vi "Results to Waveforms (array of U8).vi"(1 "data type":u8[][](array[numeric]), 7 "result references":T1[](array[typedef]), 11 "error in (no error)":errorcluster) -> (6 "signals out":u8[][](array[numeric]), 8 "result references out":T1[](array[typedef]), 15 "error out":errorcluster)   [LabVIEW 2020, in "NI_DataFinder.lvlib"]
doc: "Extracts the signals from the results of a DataFinder search."
uses:
  <vilib>/DataFinder/NI_DataFinder.lvlib
  <vilib>/userdefined/DFSearchResult.ctl
  <vilib>/userdefined/NI_DataFinder Controls.lvlib
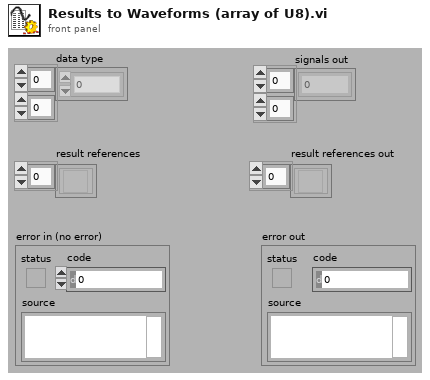
[diagram p1: front panel]
types:
  T1 = typedef "NI_DataFinder Controls.lvlib/DFSearchResult.ctl" = refnum<k20>
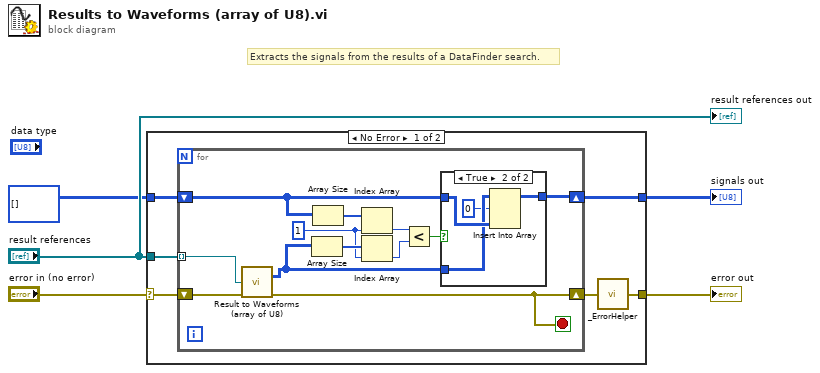
[diagram p0: block diagram]
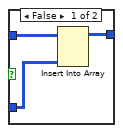
[diagram p2: hidden frame]
diagram:
  # "Extracts the signals from the results of a DataFinder search."
  n1 = case shown="No Error" "error in (no error)" {
    selector: "error in (no error)" -> [w6 w31]
    tunnel: "result references" -> [w11 _]
    tunnel: [w10 w32] -> w4
    tunnel: [w9 w31] -> w3
    tunnel: u8[][] [] ("signals out") -> [w8 w32]
    frame No Error {
      n2 = for {
        shift-right: [w15] -> w10
        shift-left: w8 -> [w14]
        tunnel: w11 -> [w23] mode=indexing
        shift-right: [w12] -> w7
        shift-left: w6 -> [w22]
        stop <- w12 stop-if-true
        w19 = 1 ("index")
        n3 = call <vilib>:"Result to Waveforms (array of U8).vi"("result reference"=w23, "error in"=w22) -> ("signals out"=w13:u8[][], "error out"=w12:errorcluster)  [unwired: 11 in, 1 out]
        n4 = Array Size(array=w13) -> (size(s)=w20:i32[])
        n5 = Array Size(array=w14) -> (size(s)=w21:i32[])
        n6 = Index Array(array=w21, index=w19) -> (element=w17:i32)
        n7 = Index Array(array=w20, index=w19) -> (element=w18:i32)
        n8 = Less?(x=w17, y=w18) -> (x < y?=w16:bool)
        n9 = case shown="True" w16 {
          tunnel: w14 -> [w25 w30]
          tunnel: w13 -> [w26 w29]
          tunnel: [w24 w27] -> w15
          frame False {
            n10 = Insert Into Array(array=w25, new element=w26) -> (w24:u8[][])  [unwired: 2 in]
          }
          frame True {
            n11 = Insert Into Array(array=w29, index (row)=0, new element=w30) -> (w27:u8[][])  [unwired: 1 in]
          }
        }
      }
      n12 = call <vilib>:"_ErrorHelper.vi"("error IO"=w7) -> ("error out"=w9:errorcluster)
    }
    frame Error {
    }
  }
  "error out" <- w3
  "signals out" <- w4
  "result references out" <- "result references"
